vi "Operation with DLL.vi"(0 "Input1":dbl, 5 "Input 2":dbl, 7 "DLL Type":T1, 9 "Arithmetic Operation":string(combo), 11 "Error in":errorcluster) -> (4 "Output":dbl, 15 "Error out":errorcluster)   [LabVIEW 2020, in "LV Connectivity.lvlib"]
doc: "This VI is used as a implementation to test the DLL implementation of C and .NET DLL Select the DLL and the arithmentic operation to be made to execute"
uses:
  LV Connectivity.lvlib
  Typedefs/DLL Type.ctl
  C:/Users/khishore.kumar/Khishore/labview_tips_2024/src/Assignment 11/builds/LV Connectivity/.NET DLL/InteropAssembly.dll
  builds/LV Connectivity/.NET DLL/InteropAssembly.dll
  builds/LV Connectivity/My DLL/SharedLib.dll
panel:
  # "DLL IMPLEMENTATION"
  # "Instructions:\n1. Select the DLL and the arithmetic operation to \nperform and give the inputs.\n2. You can terminate execution with the help of Panel\nclose"
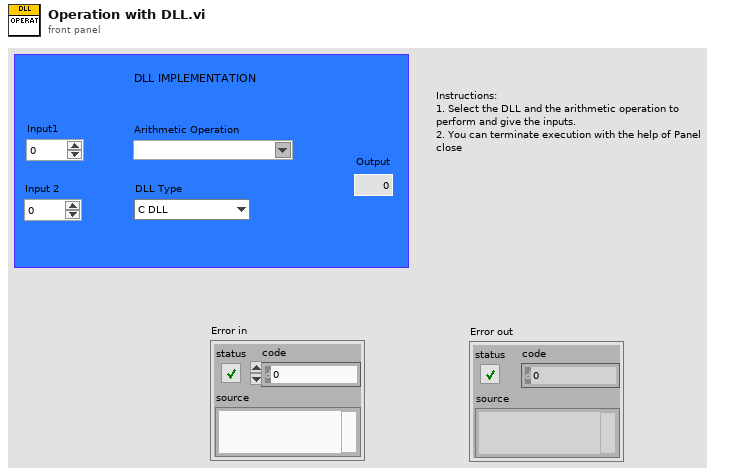
[diagram p1: front panel]
types:
  T1 = typedef "LV Connectivity.lvlib/DLL Type.ctl" = enum16{"C DLL", ".NET DLL"}
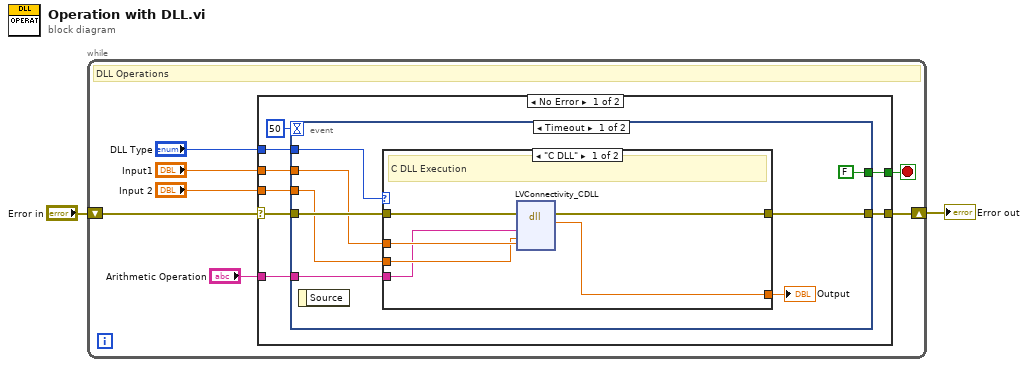
[diagram p0: block diagram]
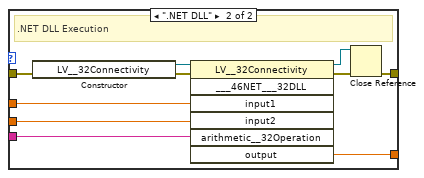
[diagram p2: hidden frame]
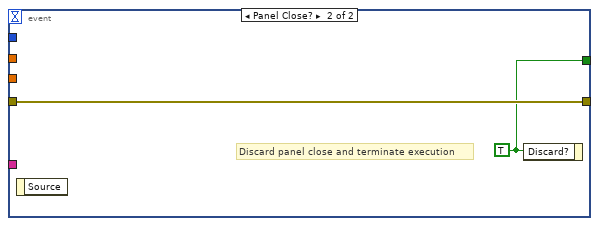
[diagram p3: hidden frame]
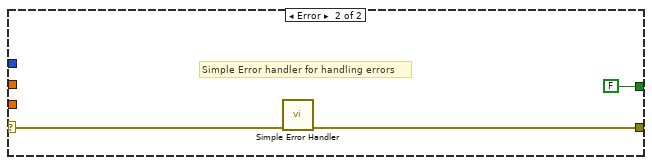
[diagram p4: hidden frame]
diagram:
  n1 = while {
    shift-right: [w9] -> w2
    shift-left: "Error in" -> [w8]
    stop <- w7 stop-if-true
    # "DLL Operations"
    n2 = case shown="No Error" w8 {
      selector: w8 -> [w17 w46]
      tunnel: [w16 w45] -> w9
      tunnel: [w15 FALSE ("Discard?")] -> w7
      tunnel: "Input1" -> [w13 _]
      tunnel: "Input 2" -> [w12 _]
      tunnel: "DLL Type" -> [w11 _]
      tunnel: "Arithmetic Operation" -> [w10 _]
      frame No Error {
        n3 = event shown="[0] Timeout" {
          selector: _ -> [_ _]
          dyn-events: _ -> [_ _]
          timeout: 50 -> [_ _]
          tunnel: w17 -> [w24 w43]
          tunnel: [w23 w43] -> w16
          tunnel: [FALSE ("Discard?") w42] -> w15
          tunnel: w13 -> [w22 _]
          tunnel: w12 -> [w21 _]
          tunnel: w11 -> [w18 _]
          tunnel: w10 -> [w20 _]
          event Timeout {
            n4 = event-data() -> ()  [unwired: 1 in, 1 out]
            n5 = case shown="\"C DLL\"" w18 {
              tunnel: w24 -> [w31 w41]
              tunnel: [w30 w36] -> w23
              tunnel: w22 -> [w28 w34]
              tunnel: w21 -> [w27 w33]
              tunnel: w20 -> [w26 w32]
              tunnel: [w29 w38] -> w19
              frame "C DLL" {
                # "C DLL Execution"
                n6 = dll-call lib="C:/Users/khishore.kumar/Khishore/labview_tips_2024/src/Assignment 11/builds/LV Connectivity/My DLL/SharedLib.dll" fn="LVConnectivity_CDLL"(error in=w31, "Arithmetic Operations"=w26, "Input2"=w27, "Input1"=w28) -> (error out=w30:errorcluster, "return type"=w29:dbl)  [unwired: 5 in, 1 out]
              }
              frame ".NET DLL" {
                # ".NET DLL Execution"
                n7 = constructor class="LV__32Connectivity"(error in=w41) -> (reference out=w40:refnum<k24>, error out=w39:errorcluster)  [unwired: 2 in, 1 out]
                n8 = invoke class="LV__32Connectivity" method="___46NET___32DLL"(reference=w40, error in=w39, "input1"=w34, "input2"=w33, "arithmetic__32Operation"=w32) -> (reference out=w35:refnum<k24>, error out=w37:errorcluster, "output"=w38:dbl)  [unwired: 2 in, 4 out]
                n9 = Close Reference(reference=w35, error in (no error)=w37) -> (error out=w36:errorcluster)
              }
            }
            "Output" <- w19
          }
          event Panel Close? {
            w42 = TRUE ("Discard?")
            # "Discard panel close and terminate execution"
            n10 = event-data() -> ()  [unwired: 1 in, 1 out]
            n11 = event-data("Discard?"=w42) -> ()  [unwired: 1 in, 1 out]
          }
        }
      }
      frame Error {
        # "Simple Error handler for handling errors"
        n12 = call <vilib>:"Simple Error Handler.vi"("error in (no error)"=w46) -> ("error out"=w45:errorcluster)  [unwired: 4 in, 4 out]
      }
    }
  }
  "Error out" <- w2
